vi "Broadcast Console.vi"(7 "name":string="BroadcastConsole") -> ()   [LabVIEW 2017, in "DebugConsole.lvlib"]
doc: "CSM Debug Console, you can use this tool:\n\n1. Select an existing CSM instance, open the front panel and block diagram.\n2. Scan the API interfaces of existing CSM instances.\n3. Select an API interface, call synchronously or asynchronously, view the return value.\n4. View the overall program's running log."
uses:
  DebugConsole.lvlib
  _Support/Typedef/_CSM_GlobalLog_MSG.ctl
  _Support/Typedef/_CSM_Response Source Message.ctl
  _Support/Typedef/_CSM_GlobalLog_MSG_TYPE.ctl
  _Support/Typedef/_CSM_List Module Scope.ctl
  _BroadcastDef.ctl
  AdvanceAPI/CSM - Broadcast Message Type.ctl
  AdvanceAPI/CSM - Convert Error to Argument.vi
  _Support/GlobalEvent/GEvt-Generate with Rule Check.vi
  AdvanceAPI/CSM - Keywords.vi
  AdvanceAPI/CSM - Make String Arguments Safe.vi
  _csmlite/_PassAllowedMessage - MsgList.vi
  _Support/GlobalEvent/Cache-GEvt Refs.vi
  _Support/GlobalEvent/LogFilter/LogFilter - Check.vi
  _Polymophic/Build Status Broadcast Message.vi
  _Polymophic/Build Interrupt Broadcast Message.vi
  _Support/GlobalEvent/LogFilter/LogFilter.lvclass
  Communicable State Machine.lvlib
  _Shared/CSM Shared.lvlib
  _ui/csm-ui-support.lvlib
  _csmlite/_csmlite.lvlib
  _csmHelper/API with lvcsm Support/CSM-Helper API with lvcsm Support.lvlib
panel:
  in  "CSM":string
  in  "List":string(combo)
  in  "Refresh API":bool
  in  "MsgString":string(combo)
  in  "-><status>":bool
  in  "-><interrupt>":bool
  in  "Arguments":string
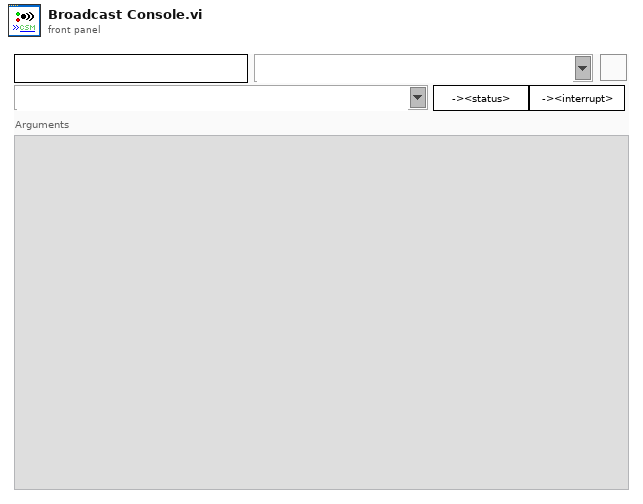
[diagram p1: front panel]
types:
  T1 = enum32{"Invalid", "Standard", "Closed", "Hidden", "Minimized", "Maximized"}
  T2 = enum32{"invalid app kind", "Development System", "Run Time System", "Student Edition", "Embedded LabVIEW", "Evaluation", "Custom"}
  T3 = typedef "Communicable State Machine.lvlib/_CSM_List Module Scope.ctl" = enum16{"Normal", "System Only", "All"}
  T4 = typedef "DebugConsole.lvlib/_BroadcastDef.ctl" = enum16{"<no action>", "Macro: Exit", "CSM: Module List Changed", "CSM: Scripts Changed", "CSM: Registration Changed", "CSM: Module Selected", "CSM: Message Excuted", "CSM: Broadcast Excuted", "CSM: Registration Action Excuted", "UI: Try to Change Command"}
  T5 = typedef "Communicable State Machine.lvlib/CSM - Broadcast Message Type.ctl" = enum16{"<Null>", "Status", "Interrupt"}
  T6 = enum8{"Enabled", "Disabled", "Disabled and Grayed Out"}
  T7 = cluster{"Shift":bool, "Ctrl":bool, "Alt":bool, "Cmd":bool, "Opt":bool}
  T8 = cluster{"Core":cluster{"Current VI Reference":refnum<vi>, "Close Panel on Exit?":bool}, "CSM Global Log Event":refnum<user-event>, "Toobar.advance":refnum<vi>[], "CSM Check History":string[], "History Length":i32}
  T9 = cluster{"Current VI Reference":refnum<vi>, "Close Panel on Exit?":bool}
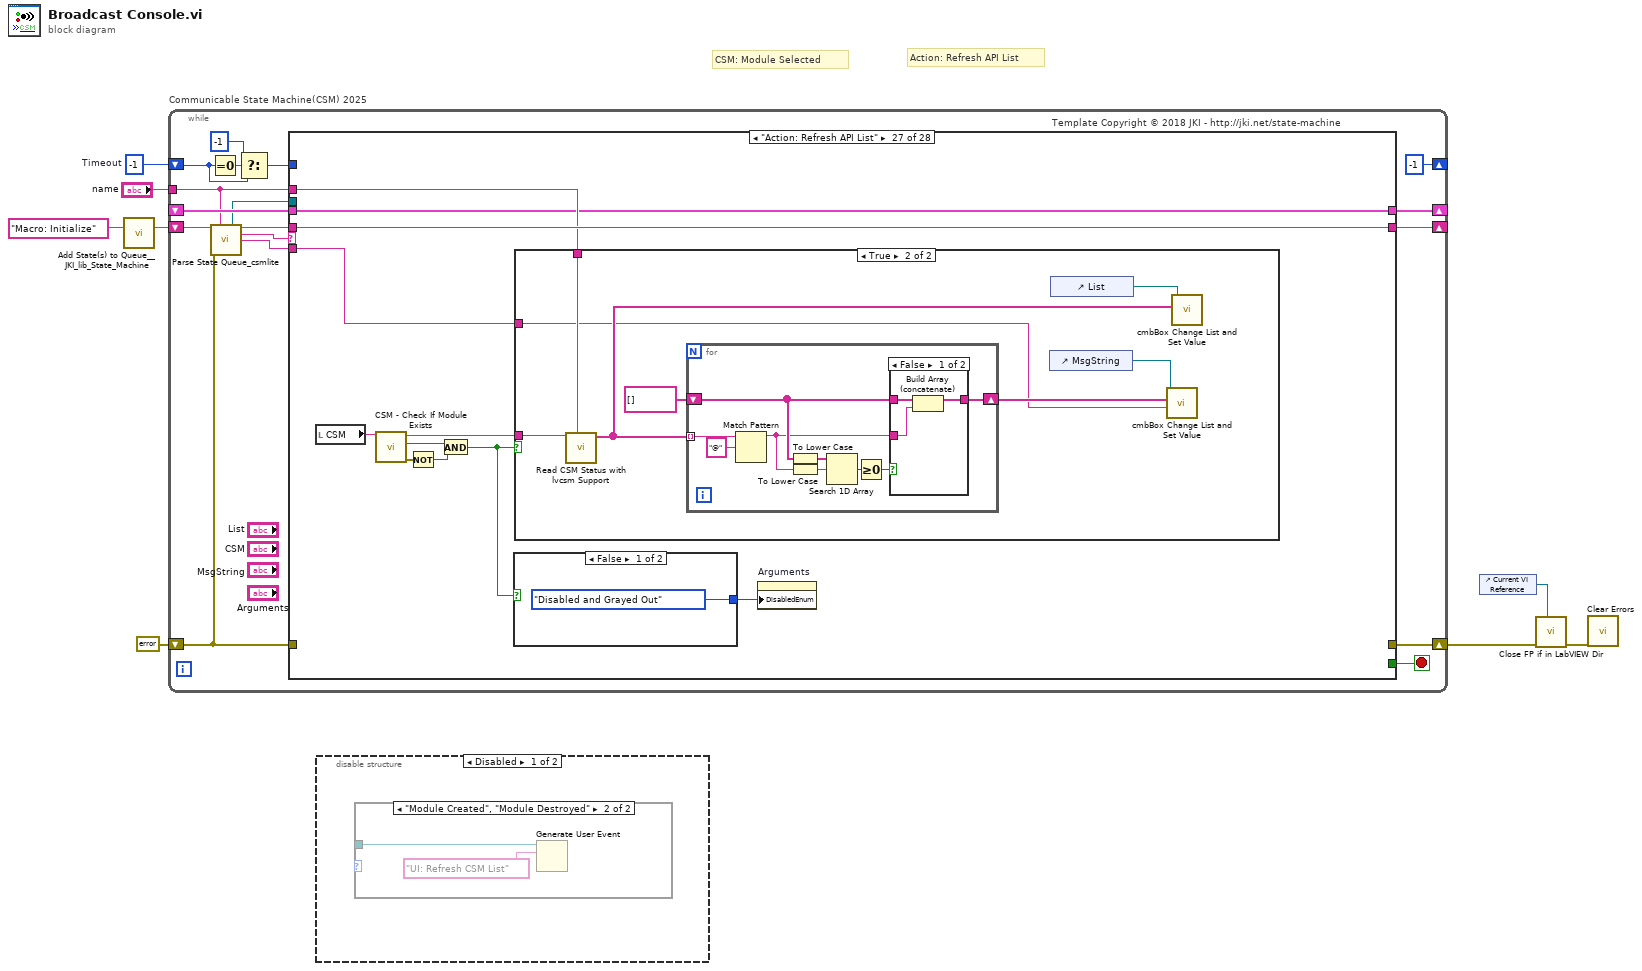
[diagram p0: block diagram]
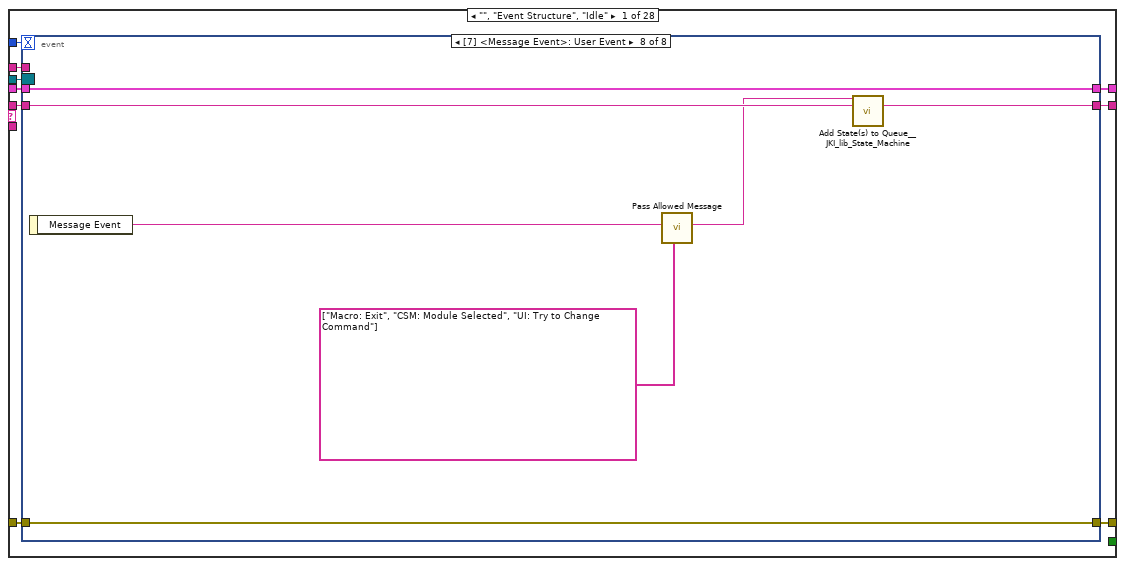
[diagram p4: hidden frame]
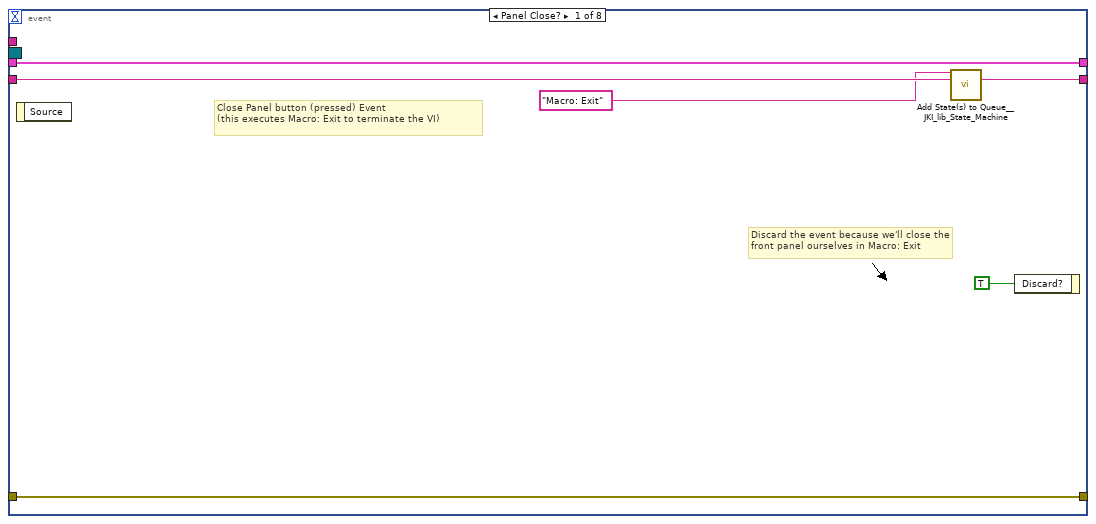
[diagram p5: hidden frame]
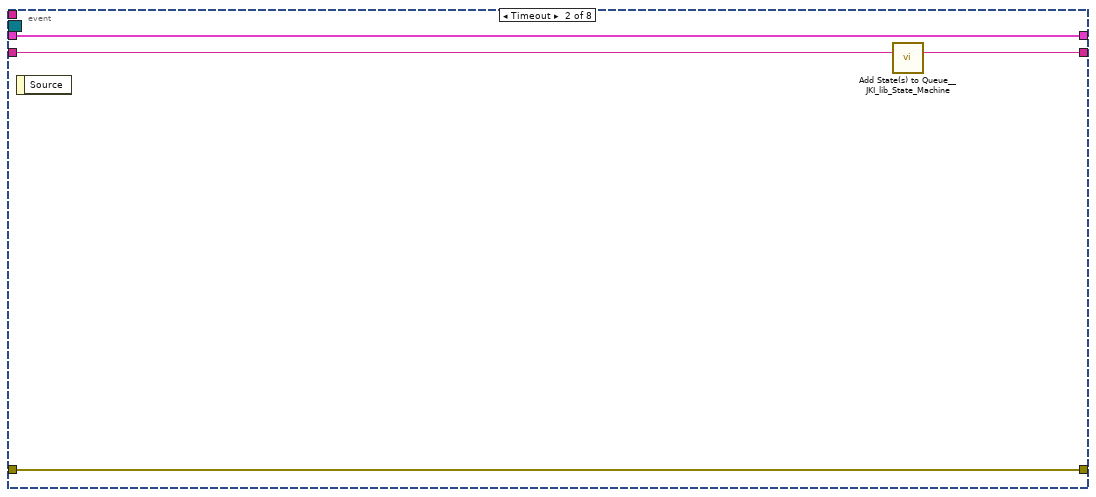
[diagram p6: hidden frame]
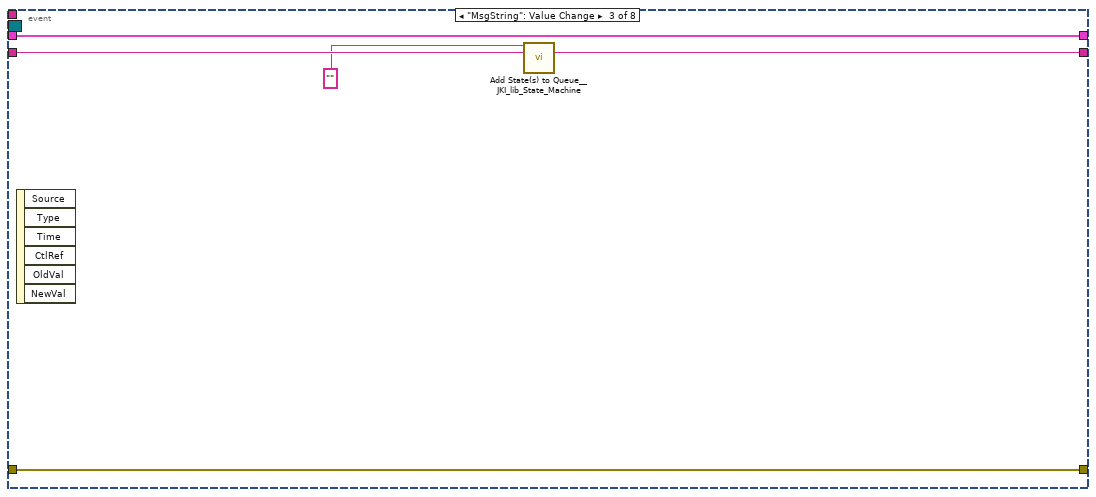
[diagram p7: hidden frame]
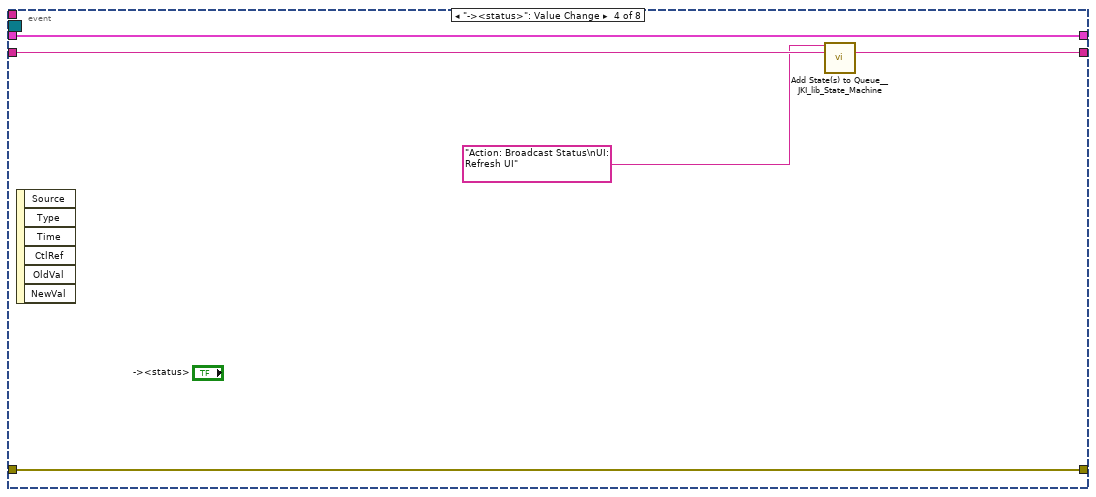
[diagram p8: hidden frame]
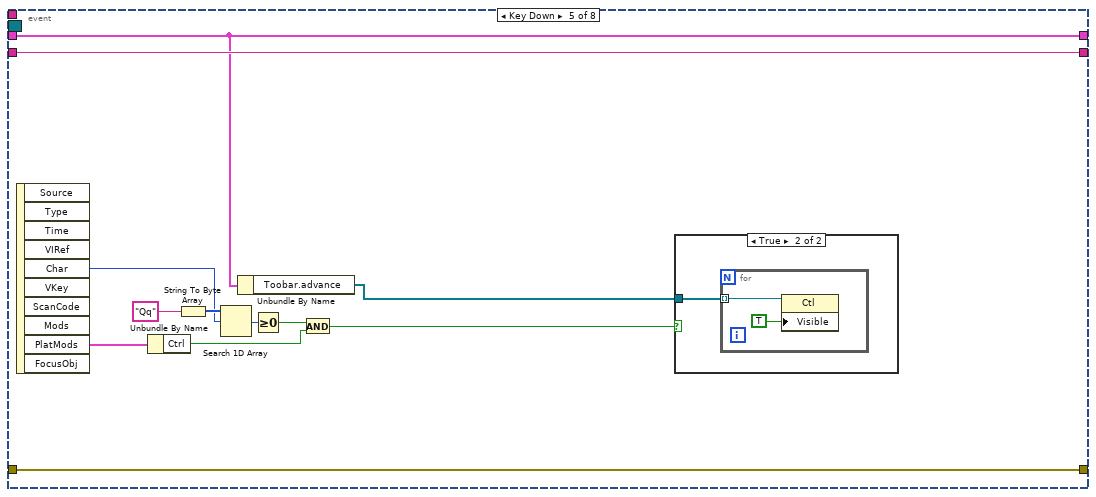
[diagram p9: hidden frame]
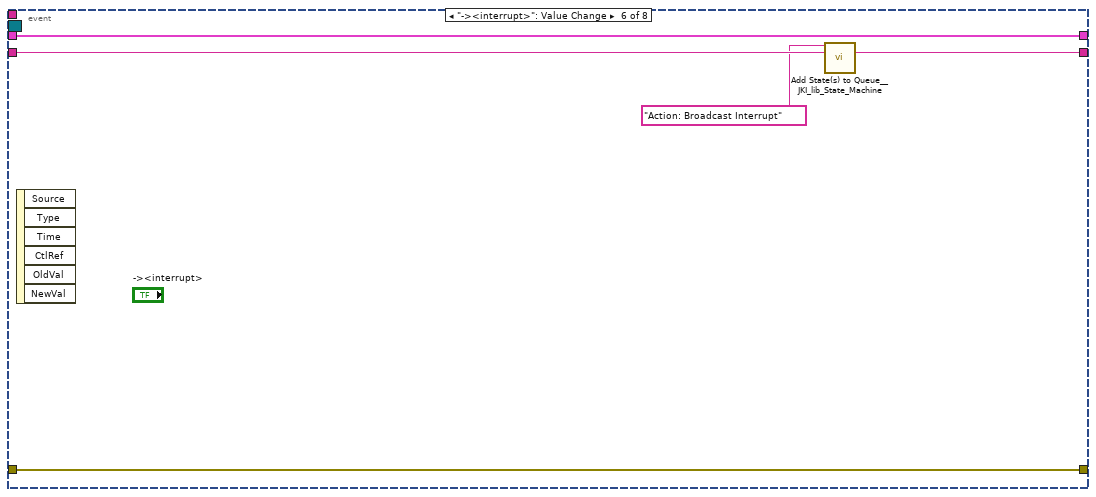
[diagram p11: hidden frame]
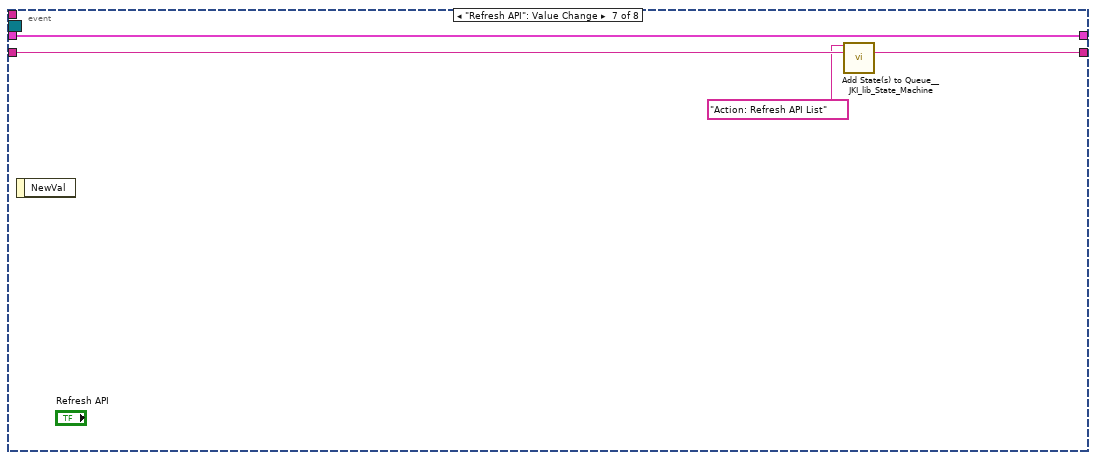
[diagram p12: hidden frame]
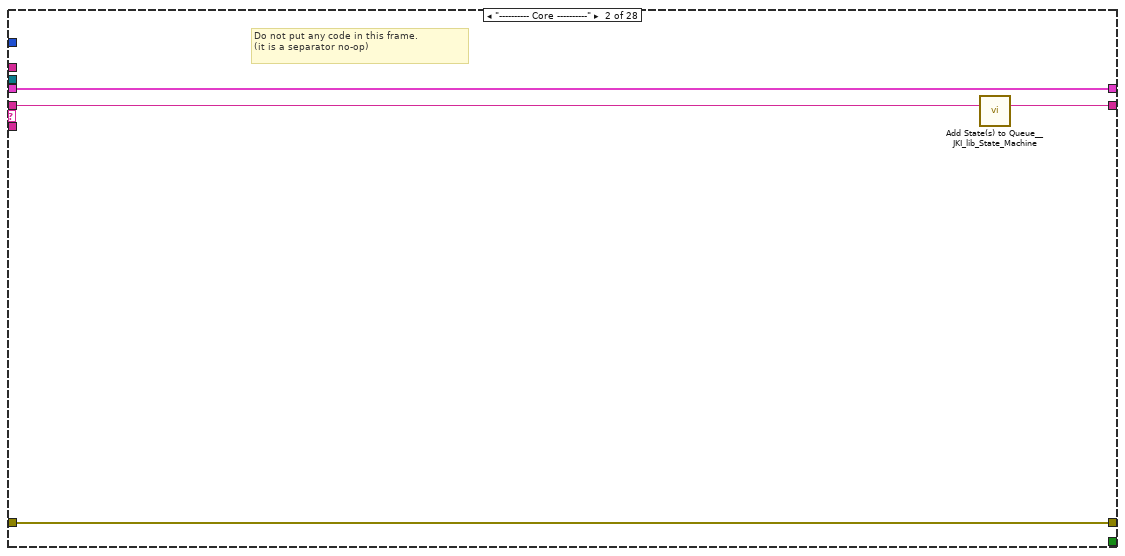
[diagram p13: hidden frame]
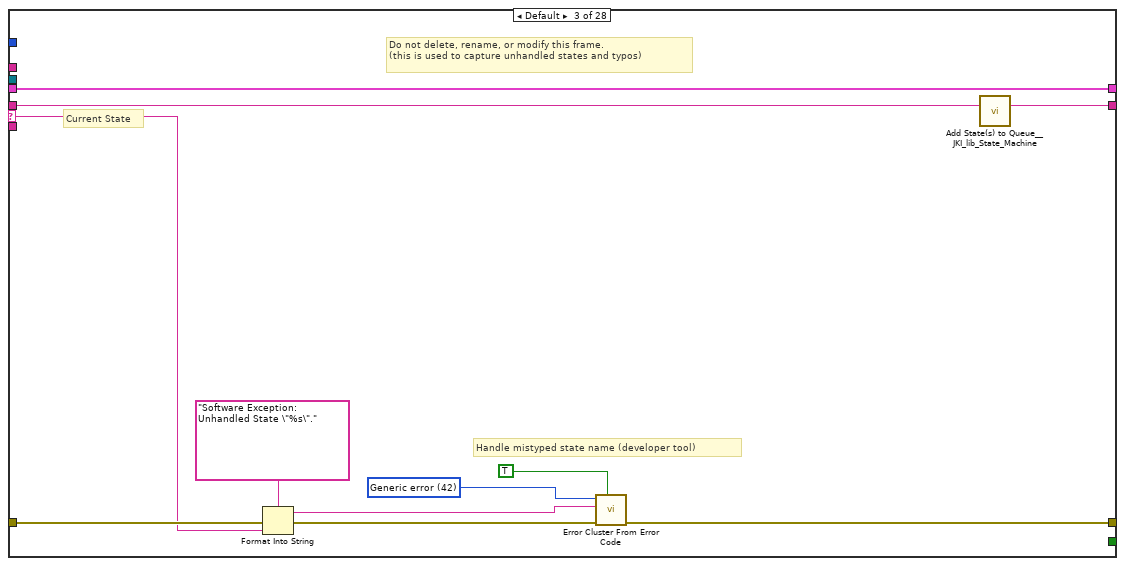
[diagram p14: hidden frame]
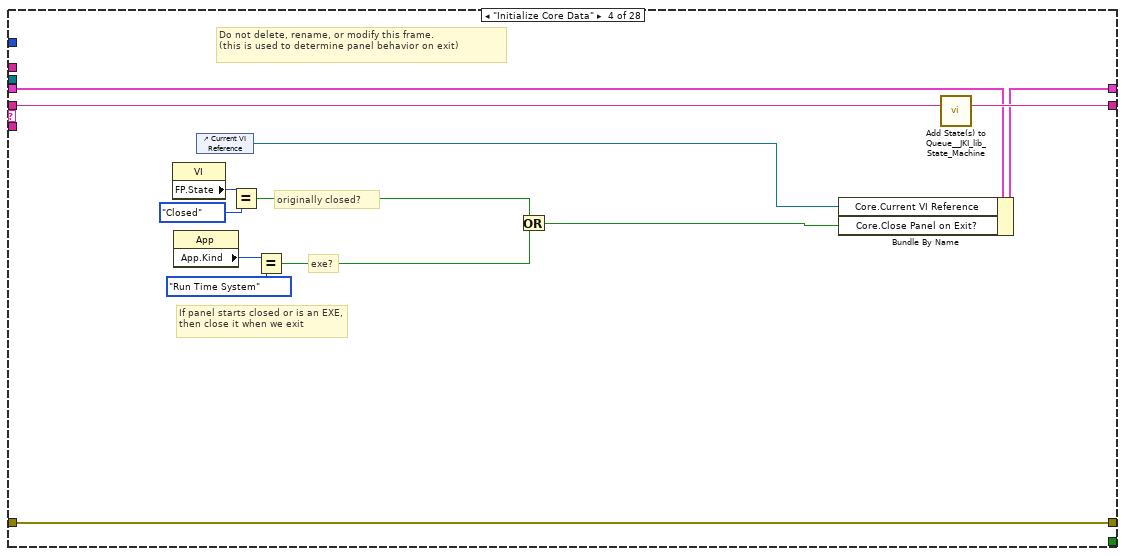
[diagram p15: hidden frame]
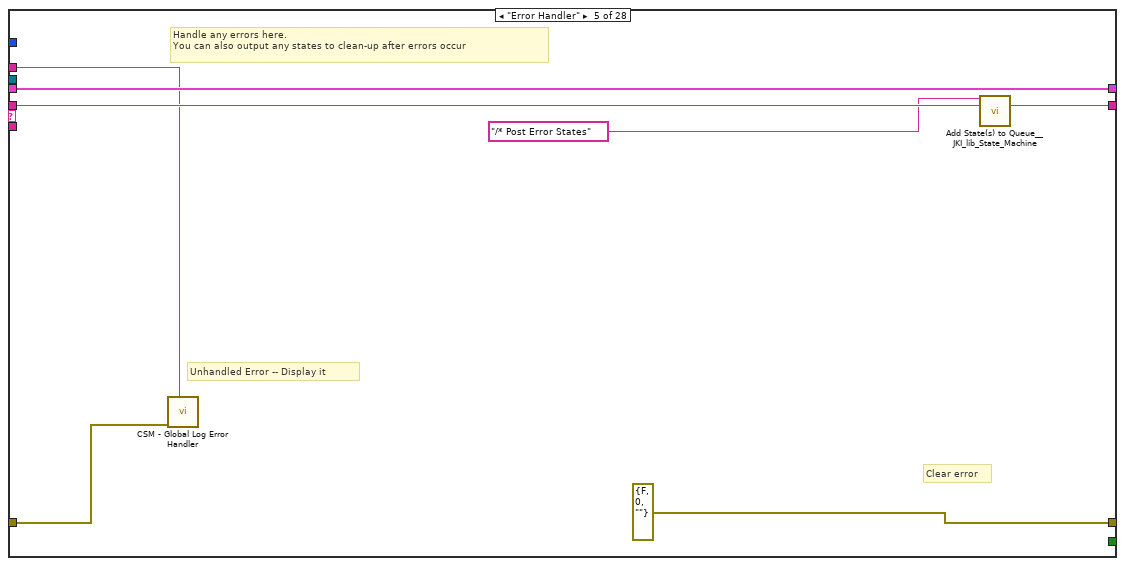
[diagram p16: hidden frame]
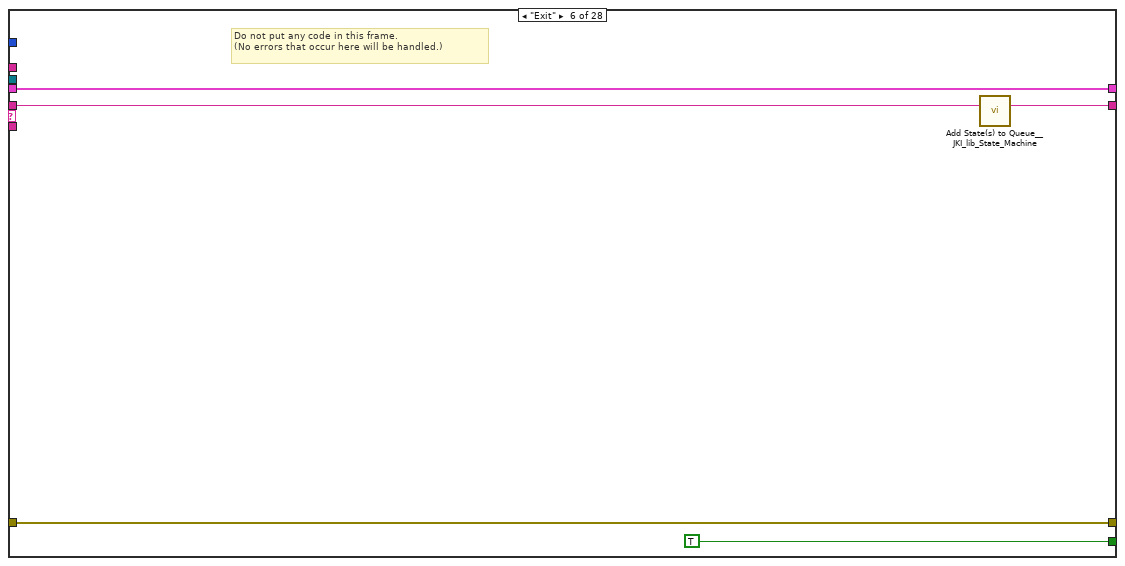
[diagram p17: hidden frame]
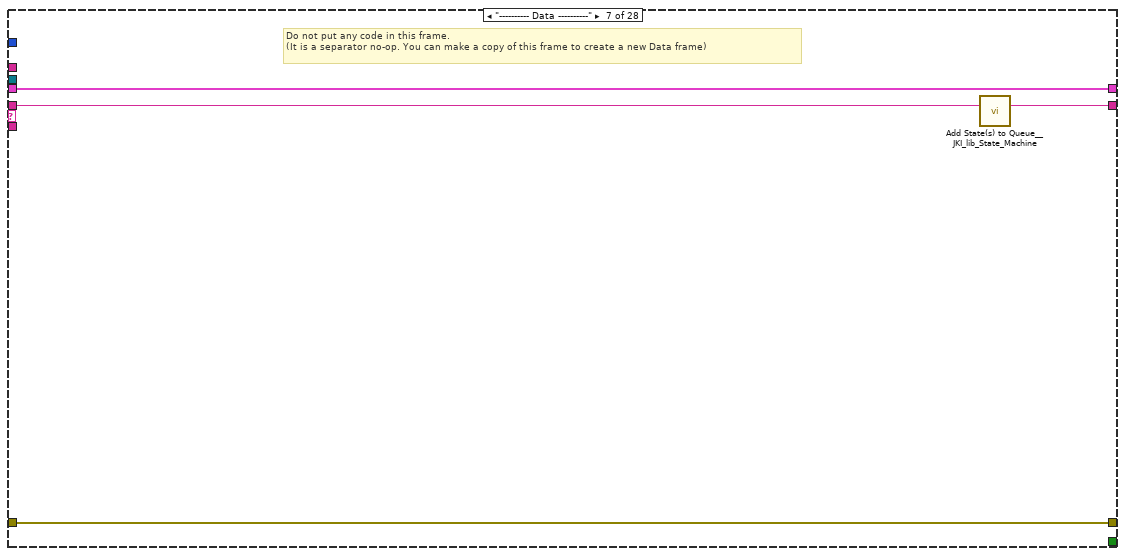
[diagram p18: hidden frame]
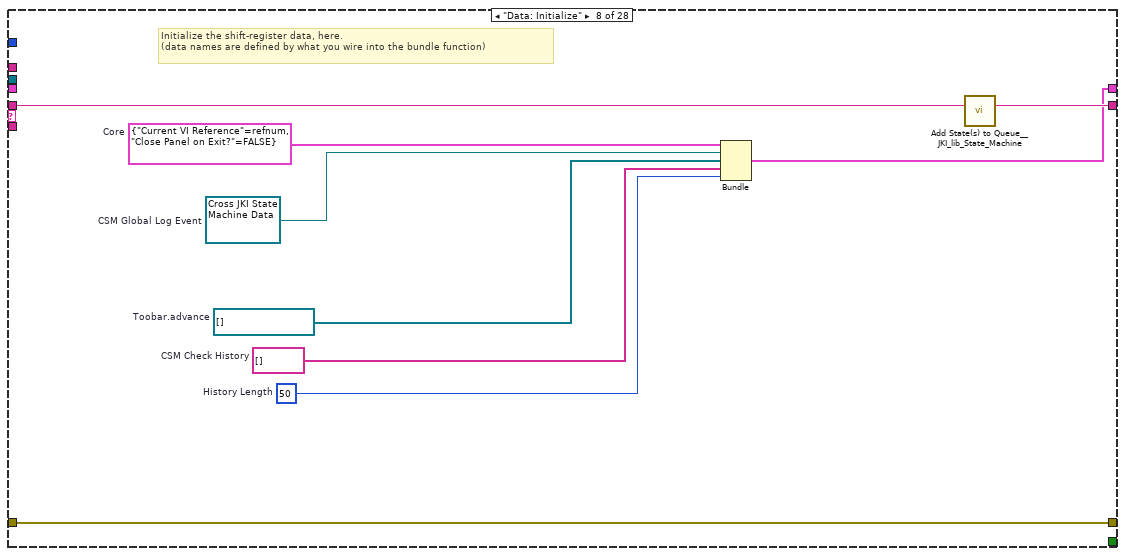
[diagram p19: hidden frame]
diagram:
  w6 = -1  # Timeout
  # "Action: Refresh API List"
  # "CSM: Module Selected"
  n1 = call <vilib>:"Add State(s) to Queue__JKI_lib_State_Machine.vi"("State(s) in (\"\")"="Macro: Initialize") -> ("States Out"=w7:string)  [unwired: 14 in]
  n2 = while "Communicable State Machine(CSM) 2025" {
    shift-right: [w18] -> _
    shift-left: _ -> [w17]
    shift-right: [w21] -> w3
    shift-left: errorcluster {"status"=FALSE, "code"=0, "source"=""} ("error out") -> [w16]
    shift-right: [w20] -> _
    shift-left: w7 -> [w22]
    tunnel: "name" -> [w10]
    shift-right: [-1 ("Timeout")] -> _
    shift-left: w6 -> [w13]
    stop <- w19 stop-if-true
    # "Template Copyright © 2018 JKI - http://jki.net/state-machine"
    n3 = Equal To 0?(x=w13) -> (x = 0?=w15:bool)
    n4 = call "Parse State Queue_csmlite.vi"("State Queue"=w22, "Current Module(\"\" to generate an ID)"=w10, "Error In (no error)"=w16) -> ("Event Registration Refnum"=w9:refnum<event-registration>, "Remaining States"=w24:string, "Current State"=w25:string, "Arguments"=w23:string)  [unwired: 9 in]
    n5 = Select(t=-1 ("Timeout"), s=w15, f=w13) -> (s? t:f=w12:i32)
    n6 = case shown="\"Action: Refresh API List\"" w25 {
      selector: w25 -> [_ _ w90 _ _ _ _ _ _ _ _ _ _ _ _ _ _ _ _ _ _ _ _ _ _ _ _ _]
      tunnel: w24 -> [w34 w89 w94 w113 w120 w125 w129 w138 w140 w147 w151 w155 w160 w169 w180 w255 w262 w268 w271 w303 w308 w315 w319 w326 w342 w354 w366 w391]
      tunnel: w23 -> [_ _ _ _ _ _ _ _ _ _ _ _ _ w164 w174 w254 w264 _ w280 _ _ _ _ _ _ _ w356 _]
      tunnel: w17 -> [w32 w86 w92 w106 w117 w123 w126 _ w139 w142 w148 w152 w157 w167 w176 w252 w265 w267 w284 w300 w305 w312 w316 w324 w340 w353 w363 w390]
      tunnel: [w31 w87 w96 w110 errorcluster {"status"=FALSE, "code"=0, "source"=""} ("error out") w122 w127 w135 w141 w143 w149 w153 w158 w165 w177 w256 w266 w269 w285 w301 w306 w313 w317 w323 w339 w355 _ w392] -> w21
      tunnel: w16 -> [w30 w87 w95 w110 w116 w122 w127 w135 w141 w144 w149 w153 w158 w166 w178 w256 w266 w269 w285 w301 w306 w313 w317 _ _ w355 _ w392]
      tunnel: [w33 w88 w93 w112 w119 w124 w128 w137 w140 w146 w150 w154 w159 w168 w179 w255 w263 w268 w272 w302 w307 w314 w318 w325 w341 w354 w366 w391] -> w20
      tunnel: [_ _ _ _ _ TRUE _ _ _ _ _ _ _ _ _ _ _ _ _ _ _ _ _ _ _ _ _ _] -> w19
      tunnel: [w29 w86 w92 w111 w117 w123 w126 w136 w139 w142 w148 w152 w157 w167 w176 w252 w265 w267 w284 w300 w305 w312 w316 w324 w340 w353 w363 w390] -> w18
      tunnel: w12 -> [w28 _ _ _ _ _ _ _ _ _ _ _ _ _ _ _ _ _ _ _ _ _ _ _ _ _ _ _]
      tunnel: w10 -> [w27 _ _ _ w114 _ _ _ _ _ _ _ _ _ _ _ _ _ _ _ _ _ _ _ _ _ w364 _]
      tunnel: w9 -> [w26 _ _ _ _ _ _ _ _ _ _ _ _ _ _ _ _ _ _ _ _ _ _ _ _ _ _ _]
      frame "", "Event Structure", "Idle" {
        n7 = event shown="[7] <Message Event>: User Event" {
          selector: w26 -> [_ _ _ _ _ _ _ _]
          dyn-events: _ -> [_ _ _ _ _ _ _ _]
          timeout: w28 -> [_ _ _ _ _ _ _ _]
          tunnel: w34 -> [w40 w44 w46 w51 w66 w71 w76 w82]
          tunnel: [w39 w43 w47 w52 w66 w72 w77 w83] -> w33
          tunnel: w32 -> [w37 w41 w48 w53 w55 w73 w78 w84]
          tunnel: [w38 w42 w49 w54 w65 w74 _ w85] -> w31
          tunnel: w30 -> [w38 w42 w49 w54 w65 w74 _ w85]
          tunnel: [w37 w41 w48 w53 w55 w73 w78 w84] -> w29
          tunnel: w27 -> [_ _ _ _ _ _ _ _]
          event Panel Close? {
            # "Discard the event because we'll close the front panel ourselves in Macro: Exit"
            # "Close Panel button (pressed) Event\n(this executes Macro: Exit to terminate the VI)"
            n8 = event-data() -> ()  [unwired: 1 in, 1 out]
            n9 = call <vilib>:"Add State(s) to Queue__JKI_lib_State_Machine.vi"("State(s) in Front (\"\")"="Macro: Exit", "State(s) in (\"\")"=w40) -> ("States Out"=w39:string)  [unwired: 13 in]
            n10 = event-data("Discard?"=TRUE) -> ()  [unwired: 1 in, 1 out]
          }
          event Timeout {
            n11 = event-data() -> ()  [unwired: 1 in, 1 out]
            n12 = call <vilib>:"Add State(s) to Queue__JKI_lib_State_Machine.vi"("State(s) in (\"\")"=w44) -> ("States Out"=w43:string)  [unwired: 14 in]
          }
          event "MsgString": Value Change {
            n13 = event-data() -> ()  [unwired: 1 in, 6 out]
            n14 = call <vilib>:"Add State(s) to Queue__JKI_lib_State_Machine.vi"("State(s) in Front (\"\")"="" ("State(s) in Front (\"\")"), "State(s) in (\"\")"=w46) -> ("States Out"=w47:string)  [unwired: 13 in]
          }
          event "-><status>": Value Change {
            n15 = event-data() -> ()  [unwired: 1 in, 6 out]
            n16 = call <vilib>:"Add State(s) to Queue__JKI_lib_State_Machine.vi"("State(s) in Front (\"\")"="Action: Broadcast Status\nUI: Refresh UI" ("State(s) in Front (\"\")"), "State(s) in (\"\")"=w51) -> ("States Out"=w52:string)  [unwired: 13 in]
          }
          event Key Down {
            n17 = event-data() -> ("Char"=w56:i16, "PlatMods"=w57:T7)  [unwired: 1 in, 8 out]
            n18 = Unbundle By Name(w57) -> ("Ctrl"=w60:bool)
            n19 = String To Byte Array(string="Qq") -> (unsigned byte array=w62:u8[])
            n20 = Search 1D Array(1D array=w62, element=w56) -> (index of element=w63:i32)  [unwired: 1 in]
            n21 = Unbundle By Name(w55) -> ("Toobar.advance"=w58:refnum<vi>[])
            n22 = Greater Or Equal To 0?(x=w63) -> (x >= 0?=w64:bool)
            n23 = And(x=w64, y=w60) -> (x .and. y?=w59:bool)
            n24 = case shown="True" w59 {
              tunnel: w58 -> [_ w67]
              frame False {
              }
              frame True {
                n25 = for {
                  tunnel: w67 -> [w69] mode=indexing
                  n26 = property class="Ctl"(reference=w69, "Visible"=TRUE) -> ()  [unwired: 1 in, 2 out]
                }
              }
            }
          }
          event "-><interrupt>": Value Change {
            n27 = event-data() -> ()  [unwired: 1 in, 6 out]
            n28 = call <vilib>:"Add State(s) to Queue__JKI_lib_State_Machine.vi"("State(s) in Front (\"\")"="Action: Broadcast Interrupt" ("State(s) in Front (\"\")"), "State(s) in (\"\")"=w71) -> ("States Out"=w72:string)  [unwired: 13 in]
          }
          event "Refresh API": Value Change {
            n29 = event-data() -> ()  [unwired: 1 in, 1 out]
            n30 = call <vilib>:"Add State(s) to Queue__JKI_lib_State_Machine.vi"("State(s) in Front (\"\")"="Action: Refresh API List" ("State(s) in Front (\"\")"), "State(s) in (\"\")"=w76) -> ("States Out"=w77:string)  [unwired: 13 in]
          }
          event User Event {
            n31 = event-data() -> ("Message Event"=w81:string)  [unwired: 1 in]
            n32 = call-poly "Pass Allowed Message.vi"("Allowed Message"=string[] ["Macro: Exit", "CSM: Module Selected", "UI: Try to Change Command"], "JKISM External Event"=w81) -> ("States"=w80:string)  [unwired: 7 in]
            n33 = call <vilib>:"Add State(s) to Queue__JKI_lib_State_Machine.vi"("State(s) in Front (\"\")"=w80, "State(s) in (\"\")"=w82) -> ("States Out"=w83:string)  [unwired: 13 in]
          }
        }
      }
      frame "---------- Core ----------" {
        # "Do not put any code in this frame.\n(it is a separator no-op)"
        n34 = call <vilib>:"Add State(s) to Queue__JKI_lib_State_Machine.vi"("State(s) in (\"\")"=w89) -> ("States Out"=w88:string)  [unwired: 14 in]
      }
      frame Default {
        w99 = 42 items=["No error", "Argument error", "Memory is full", "Out of zone", "End of file", "File already open", "Generic file I/O error", "File not found", "File permission error", "Disk is full", "Duplicate path", "Too many files open", "System feature not enabled", "Resource file not found", "Cannot add resource", "Resource not found", "Image not found", "Image memory error", "Pen does not exist", "Config type invalid", "Config token not found", "Config parse error", "Config memory error", "Bad external code format", "Bad external code offset", "External code not present", "Null window", "Destroy window error", "Null menu", "Print aborted", "Bad print record", "Print driver error", "Windows error during printing", "Memory error during printing", "Print dialog error", "Generic print error", "Invalid device refnum", "Device not found", "Device parameter error", "Device unit error", "Cannot open device", "Device call aborted", "Generic error", "Cancelled by user", "Object ID too low", "Object ID too high", "Object not in heap", "Unknown heap", "Unknown object (invalid DefProc)", "Unknown object (DefProc not in table)", "Message out of range", "Invalid (null) method", "Unknown message", "Manager call not supported", "Bad address", "Network operation in progress", "Network operation timed out", "Connection is busy", "Network attribute not supported", "Network error", "Address in use", "System out of memory", "Connection aborted", "Connection refused", "Not connected", "Already connected", "Connection closed", "Initialization error (interapplication manager)", "Bad occurrence", "Wait on unbound occurrence handler", "Occurrence queue overflow", "Datalog type conflict", "Unused", "Unrecognized type (interapplication manager)", "Memory corrupt", "Failed to make temporary DLL", "Old CIN version", "Drag socket not found", "Failed to load drop-object", "Failed to register OLE object", "Failed to release OLE object", "Format specifier type mismatch", "Unknown format specifier", "Too few format specifiers", "Too many format specifiers", "Scan failed", "Newer CIN version", "Error converting to variant", "Runtime menu error", "Password tampered", "Variant attribute not found", "Incompatible variant data type", "Event data is not available", "Event Store is not present", "Occurrence is not found", "Event Queue is not created", "Event info is not available", "Refnum passed is NULL", "Error retrieving Class GUID", "Error retrieving CoClass GUID", "Error retrieving TypeLib GUID.", "Bad built application magic bytes.", "Specific driver is different from the specific driver associated with the Logical Name.", "There is no session opened to the class driver.", "Max Error", "MAX - Error with config objects", "MAX - Error loading configuration", "MAX - Group not supported"]
        # "Current State"
        # "Do not delete, rename, or modify this frame.\n(this is used to capture unhandled states and typos)"
        # "Handle mistyped state name (developer tool)"
        n35 = Format Into String(format string="Software Exception: Unhandled State \"%s\"." ("message"), error in=w95, w90) -> (resulting string=w98:string, error out=w97:errorcluster)  [unwired: 1 in]
        n36 = call <vilib>:"Error Cluster From Error Code.vi"("show call chain? (False)"=TRUE, "error in (no error)"=w97, "error message (\"\")"=w98, "error code (0)"=w99) -> ("error out"=w96:errorcluster)  [unwired: 5 in]
        n37 = call <vilib>:"Add State(s) to Queue__JKI_lib_State_Machine.vi"("State(s) in (\"\")"=w94) -> ("States Out"=w93:string)  [unwired: 14 in]
      }
      frame "Initialize Core Data" {
        # "Do not delete, rename, or modify this frame.\n(this is used to determine panel behavior on exit)"
        # "originally closed?"
        # "exe?"
        # "If panel starts closed or is an EXE, then close it when we exit"
        n38 = property class="VI"() -> ("FP.State"=w103:T1)  [unwired: 2 in, 2 out]
        n39 = property class="App"() -> ("App.Kind"=w109:T2)  [unwired: 2 in, 2 out]
        n40 = control-ref of="Current VI Reference"() -> (w104:refnum<vi>)
        n41 = Equal?(x=w103, y=T1."Closed" ("Front Panel Window:State")) -> (x = y?=w101:bool)
        n42 = Equal?(x=w109, y=T2."Run Time System" ("Application:Kind")) -> (x = y?=w107:bool)
        n43 = Or(x=w101, y=w107) -> (x .or. y?=w105:bool)
        n44 = Bundle By Name(cluster=w106, "Core.Current VI Reference"=w104, "Core.Close Panel on Exit?"=w105) -> (w111:T8)
        n45 = call <vilib>:"Add State(s) to Queue__JKI_lib_State_Machine.vi"("State(s) in (\"\")"=w113) -> ("States Out"=w112:string)  [unwired: 14 in]
      }
      frame "Error Handler" {
        # "Unhandled Error -- Display it"
        # "Handle any errors here.\nYou can also output any states to clean-up after errors occur"
        # "Clear error"
        n46 = call "CSM - Global Log Error Handler.vi"("Place (\"\" to Use VI's Name)"=w114, "Error In"=w116) -> ()  [unwired: 9 in, 1 out]
        n47 = call <vilib>:"Add State(s) to Queue__JKI_lib_State_Machine.vi"("State(s) in Front (\"\")"="/* Post Error States", "State(s) in (\"\")"=w120) -> ("States Out"=w119:string)  [unwired: 13 in]
      }
      frame "Exit" {
        # "Do not put any code in this frame.\n(No errors that occur here will be handled.)"
        n48 = call <vilib>:"Add State(s) to Queue__JKI_lib_State_Machine.vi"("State(s) in (\"\")"=w125) -> ("States Out"=w124:string)  [unwired: 14 in]
      }
      frame "---------- Data ----------" {
        # "Do not put any code in this frame.\n(It is a separator no-op. You can make a copy of this frame to create a new Data frame)"
        n49 = call <vilib>:"Add State(s) to Queue__JKI_lib_State_Machine.vi"("State(s) in (\"\")"=w129) -> ("States Out"=w128:string)  [unwired: 14 in]
      }
      frame "Data: Initialize" {
        w130 = 50  # History Length
        w131 = string[] []  # CSM Check History
        w132 = refnum<vi>[] []  # Toobar.advance
        w133 = refnum<user-event> refnum  # CSM Global Log Event
        w134 = T9 {"Current VI Reference"=refnum, "Close Panel on Exit?"=FALSE}  # Core
        # "Initialize the shift-register data, here.\n(data names are defined by what you wire into the bundle function)"
        n50 = Bundle("Core"=w134, "CSM Global Log Event"=w133, "Toobar.advance"=w132, "CSM Check History"=w131, "History Length"=w130) -> (w136:T8)  [unwired: 1 in]
        n51 = call <vilib>:"Add State(s) to Queue__JKI_lib_State_Machine.vi"("State(s) in (\"\")"=w138) -> ("States Out"=w137:string)  [unwired: 14 in]
      }
      frame "Data: Initialize References" {
      }
      frame "Data: Cleanup" {
        # "Cleanup any data and references, here.\n(this is called automatically, by the Macro: Exit)"
        n52 = Unbundle By Name(w142) -> ("Core.Current VI Reference"=w145:refnum<vi>)
        n53 = Close Reference(reference=w145, error in (no error)=w144) -> (error out=w143:errorcluster)
        n54 = call <vilib>:"Add State(s) to Queue__JKI_lib_State_Machine.vi"("State(s) in (\"\")"=w147) -> ("States Out"=w146:string)  [unwired: 14 in]
      }
      frame "---------- Events ----------" {
        # "Do not put any code in this frame.\n(It is a separator no-op. You can make a copy of this frame to create a new UI frame)"
        n55 = call <vilib>:"Add State(s) to Queue__JKI_lib_State_Machine.vi"("State(s) in (\"\")"=w151) -> ("States Out"=w150:string)  [unwired: 14 in]
      }
      frame "---------- UI ----------" {
        # "Do not put any code in this frame.\n(It is a separator no-op. You can make a copy of this frame to create a new UI frame)"
        n56 = call <vilib>:"Add State(s) to Queue__JKI_lib_State_Machine.vi"("State(s) in (\"\")"=w155) -> ("States Out"=w154:string)  [unwired: 14 in]
      }
      frame "UI: Initialize" {
        # "Initialize the User Interface, here.\n(this is called automatically, by the Macro: Init)"
        n57 = Unbundle By Name(w157) -> ("Toobar.advance"=w156:refnum<vi>[])
        n58 = disable-structure shown="Disabled" {
          disable-tunnel: w156 -> [w161 _]
          frame Disabled {
            n59 = for {
              tunnel: w161 -> [w163] mode=indexing
              n60 = property class="Ctl"(reference=w163, "Visible"=FALSE) -> ()  [unwired: 1 in, 2 out]
            }
          }
          frame Enabled {
          }
        }
        n61 = call <vilib>:"Add State(s) to Queue__JKI_lib_State_Machine.vi"("State(s) in (\"\")"=w160) -> ("States Out"=w159:string)  [unwired: 14 in]
      }
      frame "UI: Cursor Set" {
        # "Argument"
        # "Set and Unset Cursor Busy.\n(Usage: \"UI: Cursor Set >> Busy|Idle\")"
        n62 = case shown="\"Idle\", Default" w164 {
          tunnel: w166 -> [w171 w173]
          tunnel: [w170 w172] -> w165
          frame "Idle", Default {
            n63 = call <vilib>:"Unset Busy.vi"("error in (no error)"=w171) -> ("error out"=w170:errorcluster)  [unwired: 10 in]
          }
          frame "Busy" {
            n64 = call <vilib>:"Set Busy.vi"("error in (no error)"=w173) -> ("error out"=w172:errorcluster)  [unwired: 9 in, 1 out]
          }
        }
        n65 = call <vilib>:"Add State(s) to Queue__JKI_lib_State_Machine.vi"("State(s) in (\"\")"=w169) -> ("States Out"=w168:string)  [unwired: 14 in]
      }
      frame "UI: Front Panel State" {
        # "Argument"
        # "Set Front Panel Open or Closed\n(Usage: \"UI: Front Panel State >> Open|Close\")"
        n66 = Unbundle By Name(w176) -> ("Core.Current VI Reference"=w175:refnum<vi>)
        n67 = case shown="\"Minimize\", \"Minimized\"" w174 {
          tunnel: w178 -> [w186 w201 w212 w225 w238]
          tunnel: [w188 w202 w214 w227 w240] -> w177
          tunnel: w175 -> [w187 w199 w213 w226 w239]
          frame "Open", "Standard", Default {
            w181 = T1."Standard" ("State")
            n68 = property class="VI"(reference=w187, error in=w186) -> (reference out=w184:refnum<vi>, error out=w185:errorcluster, "FP.State"=w183:T1)
            n69 = Not Equal?(x=w183, y=w181) -> (x != y?=w182:bool)
            n70 = case shown="True" w182 {
              tunnel: [w192 w194] -> w188
              tunnel: w185 -> [w191 w194]
              tunnel: w184 -> [w190 _]
              tunnel: w181 -> [w189 _]
              frame True {
                n71 = invoke class="VI" method="FP.Open"(reference=w190, error in=w191, "Activate"=TRUE, "State"=w189) -> (error out=w192:errorcluster)  [unwired: 1 in, 4 out]
              }
              frame False {
              }
            }
          }
          frame "Close", "Closed" {
            n72 = property class="VI"(reference=w199, error in=w201) -> (reference out=w198:refnum<vi>, error out=w200:errorcluster, "FP.State"=w196:T1)
            n73 = Not Equal?(x=w196, y=T1."Closed" ("Front Panel Window:State")) -> (x != y?=w195:bool)
            n74 = case shown="True" w195 {
              tunnel: [w203 w206] -> w202
              tunnel: w200 -> [w203 w205]
              tunnel: w198 -> [_ w204]
              frame False {
              }
              frame True {
                n75 = invoke class="VI" method="FP.Close"(reference=w204, error in=w205) -> (error out=w206:errorcluster)  [unwired: 1 in, 2 out]
              }
            }
          }
          frame "Hidden", "Hide" {
            w207 = T1."Hidden" ("State")
            n76 = property class="VI"(reference=w213, error in=w212) -> (reference out=w210:refnum<vi>, error out=w211:errorcluster, "FP.State"=w209:T1)
            n77 = Not Equal?(x=w209, y=w207) -> (x != y?=w208:bool)
            n78 = case shown="True" w208 {
              tunnel: [w218 w219] -> w214
              tunnel: w211 -> [w217 w219]
              tunnel: w210 -> [w216 _]
              tunnel: w207 -> [w215 _]
              frame True {
                n79 = invoke class="VI" method="FP.Open"(reference=w216, error in=w217, "State"=w215) -> (error out=w218:errorcluster)  [unwired: 2 in, 4 out]
              }
              frame False {
              }
            }
          }
          frame "Minimize", "Minimized" {
            w220 = T1."Minimized" ("State")
            n80 = property class="VI"(reference=w226, error in=w225) -> (reference out=w223:refnum<vi>, error out=w224:errorcluster, "FP.State"=w222:T1)
            n81 = Not Equal?(x=w222, y=w220) -> (x != y?=w221:bool)
            n82 = case shown="True" w221 {
              tunnel: [w231 w232] -> w227
              tunnel: w224 -> [w230 w232]
              tunnel: w223 -> [w229 _]
              tunnel: w220 -> [w228 _]
              frame True {
                n83 = invoke class="VI" method="FP.Open"(reference=w229, error in=w230, "State"=w228) -> (error out=w231:errorcluster)  [unwired: 2 in, 4 out]
              }
              frame False {
              }
            }
          }
          frame "Maximize", "Maximized" {
            w233 = T1."Maximized" ("State")
            n84 = property class="VI"(reference=w239, error in=w238) -> (reference out=w236:refnum<vi>, error out=w237:errorcluster, "FP.State"=w235:T1)
            n85 = Not Equal?(x=w235, y=w233) -> (x != y?=w234:bool)
            n86 = case shown="True" w234 {
              tunnel: [w244 w245] -> w240
              tunnel: w237 -> [w243 w245]
              tunnel: w236 -> [w242 _]
              tunnel: w233 -> [w241 _]
              frame True {
                n87 = invoke class="VI" method="FP.Open"(reference=w242, error in=w243, "State"=w241) -> (error out=w244:errorcluster)  [unwired: 2 in, 4 out]
              }
              frame False {
              }
            }
          }
        }
        n88 = call <vilib>:"Add State(s) to Queue__JKI_lib_State_Machine.vi"("State(s) in (\"\")"=w180) -> ("States Out"=w179:string)  [unwired: 14 in]
      }
      frame "UI: Autoset Arguments" {
        n89 = call "CSM - Revert Arguments-Safe String.vi"("Safe Argument String"=w254) -> ("Origin Argument String"=w246:string)  [unwired: 8 in]
        n90 = control-ref of="CSM"() -> (w249:refnum<vi>)
        n91 = call "Remove Comments from Single-line.vi"("single-line text"=w246) -> ("single-line text without comments"=w253:string)  [unwired: 2 in]
        n92 = call "Split Single-line Message.vi"("single-line text"=w253) -> ("state"=w251:string, "args"=w250:string, "source/target"=w248:string)  [unwired: 6 in, 1 out]
        n93 = case shown="\"<interrupt>\", \"<status>\"" w248 {
          selector: w248 -> [w257 _]
          tunnel: [w257 w258] -> w247
          tunnel: w246 -> [_ w259]
          frame Default {
            (unwired) enum32{"Message", "Status"}."Message" ("Tab(Msg/Status)")
          }
          frame "<interrupt>", "<status>" {
            (unwired) enum32{"Message", "Status"}."Status" ("Tab(Msg/Status)")
            n94 = Match Pattern(string=w259, regular expression="//") -> (after substring=w258:string)  [unwired: 1 in, 3 out]
          }
        }
        n95 = local write "MsgString"(w251) -> ()
        n96 = local write "Arguments"(w250) -> ()
        n97 = property on="Property Node" class="Str"(reference=w249, "Value"=w247) -> ()  [unwired: 1 in, 2 out]
      }
      frame "CSM: Module Selected" {
        n98 = local write "CSM"(w264) -> ()
        n99 = call <vilib>:"Add State(s) to Queue__jki_lib_state_machine.vi"("State(s) in Front (\"\")"="Action: Refresh API List" ("State(s) in Front (\"\")"), "State(s) in (\"\")"=w262) -> ("States Out"=w263:string)  [unwired: 13 in]
      }
      frame "UI: Refresh UI" {
      }
      frame "UI: Try to Change Command" {
        n100 = call "CSM - Convert HexStr to Data.vi"("HEX String"=w280) -> ("Variant"=w282:variant, "error out"=w283:errorcluster)  [unwired: 7 in]
        n101 = Variant To Data(error in=w283, type="", Variant=w282) -> (data=w279:string)  [unwired: 1 out]
        n102 = Match Pattern(string=w279, regular expression="[/][/]") -> (before substring=w278:string, after substring=w276:string)  [unwired: 1 in, 2 out]
        n103 = call "Split Single-line Message.vi"("single-line text"=w278) -> ("state"=w274:string, "args"=w273:string, "source/target"=w275:string)  [unwired: 6 in, 1 out]
        n104 = case shown="\"<all>\", \"<broadcast>\", \"<interrupt>\", \"<status>\"" w275 {
          tunnel: w276 -> [_ w290]
          tunnel: w274 -> [_ w287]
          tunnel: w273 -> [_ w288]
          tunnel: [_ w286] -> w270
          frame "False", Default {
          }
          frame "<all>", "<broadcast>", "<interrupt>", "<status>" {
            n105 = call "CSM - List Modules.vi"("Scope (Normal)"=_CSM_List_Module_Scope."All") -> ("Module Names"=w292:string[])  [unwired: 9 in, 1 out]
            n106 = To Lower Case(string=w292) -> (all lower case string=w294:string[])
            n107 = To Lower Case(string=w290) -> (all lower case string=w293:string)
            n108 = Search 1D Array(1D array=w294, element=w293) -> (index of element=w291:i32)  [unwired: 1 in]
            n109 = Greater Or Equal To 0?(x=w291) -> (x >= 0?=w289:bool)
            n110 = case shown="True" w289 {
              tunnel: w288 -> [_ w299]
              tunnel: w287 -> [_ w298]
              tunnel: [_ w296] -> w286
              frame False {
              }
              frame True {
                n111 = call <vilib>:"Build State String with Arguments__JKI_lib_State_Machine.vi"("Arguments (\"\")"=w298, "State"="Action: Refresh API List") -> ("State with Arguments"=w296:string)  [unwired: 4 in]
                n112 = local write "Arguments"(w299) -> ()
              }
            }
          }
        }
        n113 = call <vilib>:"Add State(s) to Queue__jki_lib_state_machine.vi"("State(s) in Front (\"\")"=w270, "State(s) in (\"\")"=w271) -> ("States Out"=w272:string)  [unwired: 13 in]
      }
      frame "---------- Macro ----------" {
        # "Do not put any code in this frame.\n(It is a separator no-op. You can make a copy of this frame to create a new Macro frame)"
        n114 = call <vilib>:"Add State(s) to Queue__JKI_lib_State_Machine.vi"("State(s) in (\"\")"=w303) -> ("States Out"=w302:string)  [unwired: 14 in]
      }
      frame "Macro: Initialize" {
        # "Initialization Macro\n(This is called once, when the VI starts)"
        n115 = call <vilib>:"Add State(s) to Queue__JKI_lib_State_Machine.vi"("State(s) in Front (\"\")"="Data: Initialize\nData: Initialize References\nInitialize Core Data\nUI: Initialize\n//UI: Front Panel State >> Open\nAction: Refresh API List\nAction: Change Btn States", "State(s) in (\"\")"=w308) -> ("States Out"=w307:string)  [unwired: 13 in]
      }
      frame "Macro: Exit" {
        # "Exit Macro\n(This is called once, when the VI exits)"
        n116 = call "_Broadcast Message.vi"("Broadcast"=_BroadcastDef."Macro: Exit") -> ()  [unwired: 10 in, 1 out]
        n117 = call <vilib>:"Add State(s) to Queue__JKI_lib_State_Machine.vi"("State(s) at Back (\"\")"="Data: Cleanup\nExit") -> ("States Out"=w310:string)  [unwired: 14 in]
        n118 = call <vilib>:"Add State(s) to Queue__JKI_lib_State_Machine.vi"("State(s) in Front (\"\")"=w310, "State(s) in (\"\")"=w315) -> ("States Out"=w314:string)  [unwired: 13 in]
      }
      frame "---------- Action ----------" {
        # "Template Separator\n(You can make a copy of, or modify, this frame)"
        n119 = call <vilib>:"Add State(s) to Queue__JKI_lib_State_Machine.vi"("State(s) in (\"\")"=w319) -> ("States Out"=w318:string)  [unwired: 14 in]
      }
      frame "Action: Broadcast Status" {
        n120 = local read "MsgString"() -> (w320:string)
        n121 = local read "Arguments"() -> (w321:string)
        n122 = local read "CSM"() -> (w322:string)
        n123 = case shown="Default" w320 {
          selector: w320 -> [_ w332]
          tunnel: w321 -> [_ w331]
          tunnel: [_ w333] -> w323
          tunnel: w322 -> [_ w330]
          frame "" {
          }
          frame Default {
            n124 = call "CSM - Request CSM to Broadcast Status Change.vi"("Module Name"=w330, "Arguments (\"\")"=w331, "Status"=w332) -> ("error out"=w333:errorcluster)  [unwired: 8 in]
            n125 = call-poly "Build Message with Arguments++.vi"("State With Arguments"=w332, "Arguments (\"\")"=w331) -> ("CSM Message String"=w335:string)  [unwired: 13 in]
            n126 = Concatenate Strings(w335, "//" ("string"), w330) -> (w329:string)
            n127 = call "CSM - Convert Data to HexStr.vi"("Variant"=w329) -> ("HEX String (0-9,A-F)"=w328:string)  [unwired: 8 in]
            n128 = call "_Broadcast Message.vi"("Argument(\"\")"=w328, "Broadcast"=_BroadcastDef."CSM: Broadcast Excuted") -> ()  [unwired: 9 in, 1 out]
          }
        }
        n129 = call <vilib>:"Add State(s) to Queue__JKI_lib_State_Machine.vi"("State(s) in (\"\")"=w326) -> ("States Out"=w325:string)  [unwired: 14 in]
      }
      frame "Action: Broadcast Interrupt" {
        n130 = local read "MsgString"() -> (w336:string)
        n131 = local read "Arguments"() -> (w337:string)
        n132 = local read "CSM"() -> (w338:string)
        n133 = case shown="Default" w336 {
          selector: w336 -> [_ w349]
          tunnel: w337 -> [_ w348]
          tunnel: [_ w350] -> w339
          tunnel: w338 -> [_ w347]
          frame "" {
          }
          frame Default {
            n134 = call "CSM - Request CSM to Broadcast Status Change.vi"("Module Name"=w347, "Priority (\"Status\")"=CSM_-_Broadcast_Message_Type."Interrupt" ("Priority (\"Status\")"), "Arguments (\"\")"=w348, "Status"=w349) -> ("error out"=w350:errorcluster)  [unwired: 7 in]
            n135 = call-poly "Build Message with Arguments++.vi"("State With Arguments"=w349, "Arguments (\"\")"=w348) -> ("CSM Message String"=w352:string)  [unwired: 13 in]
            n136 = Concatenate Strings(w352, "//" ("string"), w347) -> (w343:string)
            n137 = call "CSM - Convert Data to HexStr.vi"("Variant"=w343) -> ("HEX String (0-9,A-F)"=w345:string)  [unwired: 8 in]
            n138 = call "_Broadcast Message.vi"("Argument(\"\")"=w345, "Broadcast"=_BroadcastDef."CSM: Broadcast Excuted") -> ()  [unwired: 9 in, 1 out]
          }
        }
        n139 = call <vilib>:"Add State(s) to Queue__JKI_lib_State_Machine.vi"("State(s) in (\"\")"=w342) -> ("States Out"=w341:string)  [unwired: 14 in]
      }
      frame "Action: Change Btn States" {
      }
      frame "Action: Refresh API List" {
        n140 = local read "CSM"() -> (w362:string)
        n141 = call "CSM - Check If Module Exists.vi"("CSM Name"=w362) -> ("error out"=w360:errorcluster, "Exist?"=w361:bool, "CSM Name (Dup)"=w365:string)  [unwired: 8 in]
        n142 = Not(x=w360) -> (.not. x?=w359:bool)
        n143 = And(x=w361, y=w359) -> (x .and. y?=w357:bool)
        n144 = case shown="False" w357 {
          tunnel: [T6."Disabled and Grayed Out" ("Disabled") T6."Enabled" ("Disabled")] -> w358
          frame False {
          }
          frame True {
          }
        }
        n145 = case shown="True" w357 {
          tunnel: w365 -> [_ w374]
          tunnel: w364 -> [_ w373]
          tunnel: w356 -> [_ w367]
          frame False {
          }
          frame True {
            n146 = call "Read CSM Status with lvcsm Support.vi"("Current Module (\"\" to Generate an ID)"=w373, "CSM Name"=w374) -> ("CSMAPI List"=w371:string[])  [unwired: 8 in, 1 out]
            n147 = for {
              tunnel: w371 -> [w383] mode=indexing
              shift-right: [w377] -> w368
              shift-left: string[] [] ("regular expression") -> [w376]
              n148 = Match Pattern(string=w383, regular expression="@") -> (before substring=w375:string)  [unwired: 1 in, 3 out]
              n149 = To Lower Case(string=w376) -> (all lower case string=w380:string[])
              n150 = To Lower Case(string=w375) -> (all lower case string=w381:string)
              n151 = Search 1D Array(1D array=w380, element=w381) -> (index of element=w379:i32)  [unwired: 1 in]
              n152 = Greater Or Equal To 0?(x=w379) -> (x >= 0?=w378:bool)
              n153 = case shown="False" w378 {
                tunnel: [w385 w387] -> w377
                tunnel: w376 -> [w386 w387]
                tunnel: w375 -> [w384 _]
                frame False {
                  n154 = Build Array (concatenate)(w386, w384) -> (w385:string[])
                }
                frame True {
                }
              }
            }
            n155 = control-ref of="MsgString"() -> (w369:refnum<vi>)
            n156 = control-ref of="List"() -> (w370:refnum<vi>)
            n157 = call "cmbBox Change List and Set Value.vi"("Current(\"\")"=w367, "Strings []"=w368, "cmbBox"=w369) -> ()  [unwired: 7 in, 2 out]
            n158 = call "cmbBox Change List and Set Value.vi"("Strings []"=w371, "cmbBox"=w370) -> ()  [unwired: 8 in, 2 out]
          }
        }
        n159 = property on="Arguments" class="Str"("DisabledEnum"=w358) -> ()  [unwired: 2 in, 2 out]
      }
      frame "No Peroidic Log over 1s" {
      }
    }
  }
  n160 = disable-structure shown="Disabled" {
    frame Disabled {
      n161 = case shown="\"Module Created\", \"Module Destroyed\"" {
        selector: _ -> [_ _]
        tunnel: _ -> [_ w394]
        frame "User Log", Default {
        }
        frame "Module Created", "Module Destroyed" {
          n162 = Generate User Event(user event=w394, event data cluster="UI: Refresh CSM List" ("State(s) in Front (\"\")")) -> ()  [unwired: 2 in, 2 out]
        }
      }
    }
    frame Enabled {
    }
  }
  n163 = control-ref of="Current VI Reference"() -> (w4:refnum<vi>)
  n164 = call "Close FP if in LabVIEW Dir.vi"("VI Refnum"=w4, "Error in"=w3) -> ("Error out"=w5:errorcluster)  [unwired: 9 in]
  n165 = call <vilib>:"Clear Errors.vi"("error in (no error)"=w5) -> ()  [unwired: 5 in, 2 out]
